vi "STOP.vi"(8 "error in (no error)":errorcluster, 11 "Stop in":refnum<class "DLOwis.lvclass">) -> (0 "error out":errorcluster, 3 "Stop out":refnum<class "DLOwis.lvclass">)   [LabVIEW 2019, in "DLOwis.lvclass"]
uses:
  DLOwis.lvclass
  C:/Users/elysium/Documents/dev/TRANCON/Classes/GeneralFunctionality/GeneralFunctionality.lvclass
  GeneralFunctionality/GeneralFunctionality.lvclass/GeneralFunctionality.ctl
  GeneralFunctionality/GeneralFunctionality.lvclass
panel:
  out "Axis state":i32
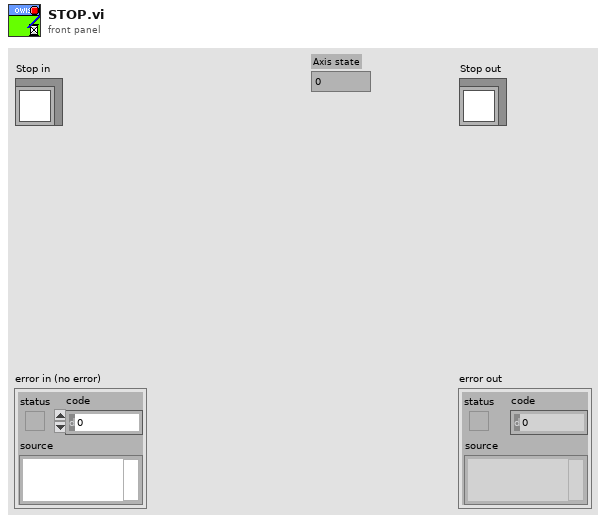
[diagram p1: front panel]
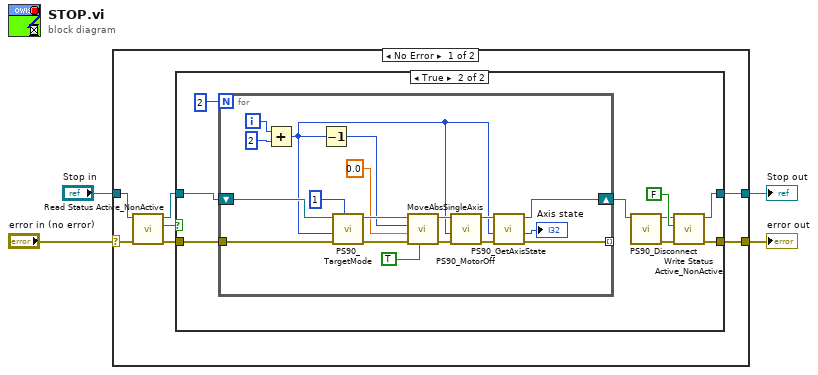
[diagram p0: block diagram]
diagram:
  n1 = case shown="No Error" "error in (no error)" {
    selector: "error in (no error)" -> [w7 w42]
    tunnel: [w11 w42] -> w2
    tunnel: [w10 w41] -> w1
    tunnel: "Stop in" -> [w9 w41]
    frame No Error {
      n2 = call "Read Status Active_NonActive.vi"("error in (no error)"=w7, "GeneralFunctionality in"=w9) -> ("error out"=w6:errorcluster, "Status Active/NonActive"=w5:bool, "GeneralFunctionality out"=w8:refnum<class "DLOwis.lvclass">)  [unwired: 7 in]
      n3 = case shown="True" w5 {
        tunnel: [w12 w21] -> w11
        tunnel: [w13 w22] -> w10
        tunnel: w8 -> [w13 w19]
        tunnel: w6 -> [w12 w18]
        frame False {
        }
        frame True {
          n4 = for {
            N: 2 -> [_]
            shift-right: [w33] -> w15
            shift-left: w19 -> [w40]
            tunnel: w18 -> [w39]
            tunnel: [w34] -> _ mode=indexing
            i -> [w37]
            n5 = Add(x=w37, y=2) -> (x+y=w25:i32)
            n6 = Decrement(x=w25) -> (x-1=w23:i32)
            n7 = call "PS90_TargetMode.vi"("Value-In"=1, "error in (no error)"=w39, "Axis number"=w25, "DLOwis.lvclass"=w40) -> ("error out"=w30:errorcluster, "DLOwis.lvclass"=w27:refnum<class "DLOwis.lvclass">)  [unwired: 3 in, 1 out]
            n8 = call-dynamic "MoveAbsSingleAxis.vi"("Wait"=TRUE, "error in (no error)"=w30, "Value"=0.0 ("dValue-In"), "Axis"=w23, "DLOwis in"=w27) -> ("error out"=w29:errorcluster, "DLOwis out"=w28:refnum<class "DLOwis.lvclass">)  [unwired: 5 in]
            n9 = call "PS90_MotorOff.vi"("error in (no error)"=w29, "Axis number"=w25, "DLOwis.lvclass"=w28) -> ("error out"=w35:errorcluster, "DLOwis.lvclass"=w32:refnum<class "DLOwis.lvclass">)  [unwired: 7 in]
            n10 = call "PS90_GetAxisState.vi"("error in (no error)"=w35, "Axis number"=w25, "DLOwis.lvclass"=w32) -> ("error out"=w34:errorcluster, "Axis state"=→"Axis state":i32, "DLOwis.lvclass"=w33:refnum<class "DLOwis.lvclass">)  [unwired: 6 in]
          }
          n11 = call "PS90_Disconnect.vi"("DLOwis.lvclass"=w15) -> ("error out"=w16:errorcluster, "DLOwis.lvclass"=w14:refnum<class "DLOwis.lvclass">)  [unwired: 5 in]
          n12 = call "Write Status Active_NonActive.vi"("error in (no error)"=w16, "Status Active/NonActive"=FALSE, "GeneralFunctionality in"=w14) -> ("error out"=w21:errorcluster, "GeneralFunctionality out"=w22:refnum<class "DLOwis.lvclass">)  [unwired: 7 in]
        }
      }
    }
    frame Error {
    }
  }
  "error out" <- w2
  "Stop out" <- w1
